vi "Emballage_Lecture_Colonne_Tablebdd.vi"(7 "Where colonne":string[](array[string]), 8 "Error in":errorcluster caption="Error in (no error)", 9 "where valeur":string[](array[string]), 10 "Table":string="configEmballage", 11 "Colonne":string) -> (0 "Error out":errorcluster, 1 "chemin complet":path, 2 "Result Set":string[][](table) caption="Result Set (from first statement with results)", 3 "Column Names":string[](array[string]))   [LabVIEW 2020]
uses:
  Modules/FS/60_FS_Controles/60_FS_SetGet.ctl
  <vilib>/drjdpowell/SQLite Library/SQL Connection/Open (path).vi
  <vilib>/drjdpowell/SQLite Library/SQL Connection/Open (string).vi
  <vilib>/AdvancedString/Path To Command Line String.vi
  <vilib>/drjdpowell/SQLite Library/SQL Connection/Connection.lvclass
panel:
  out "Chaîne":string
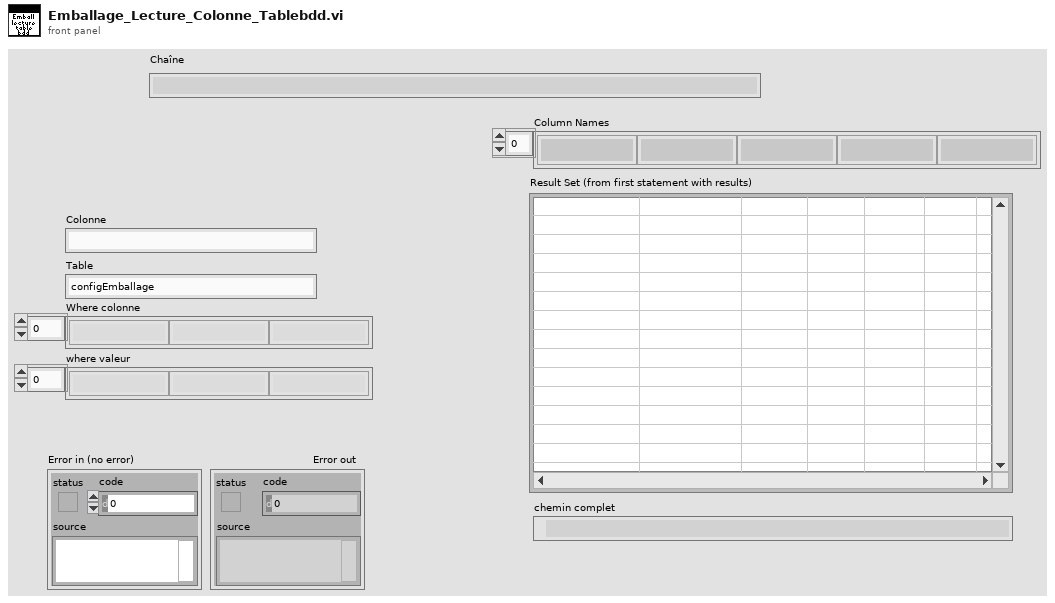
[diagram p1: front panel]
types:
  T1 = typedef "60_FS_SetGet.ctl" = enum16{"set", "get"}
  T2 = typedef "60_FS_CLT_Chemins.ctl" = cluster{"Racine_local":path, "Racine_reseau":path, "Racine_Support_Application":path, "Fichier_Journalisation":path, "Connexion_BDD_VSX":path, "Connexion_BDD_PLZ":path}
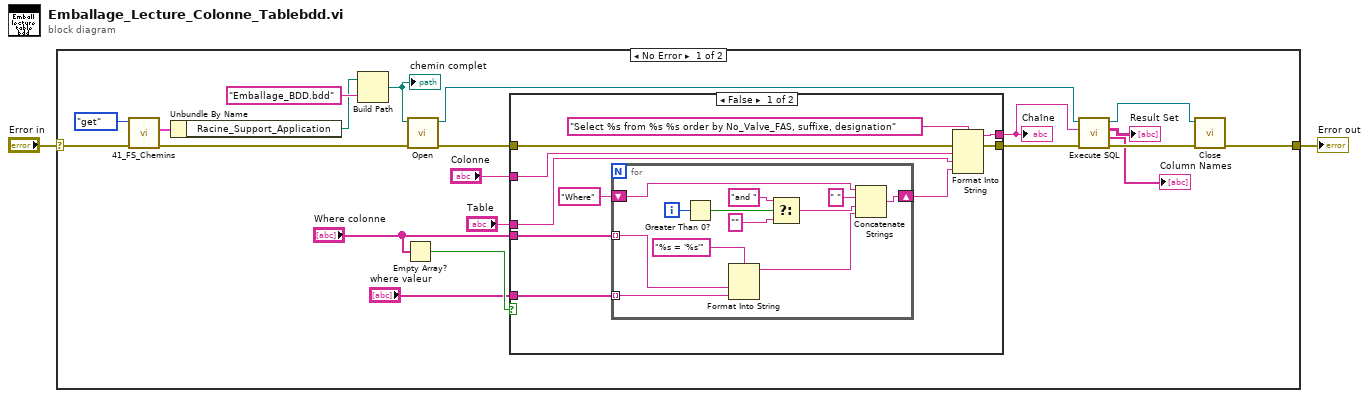
[diagram p0: block diagram]
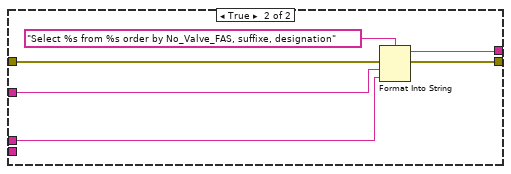
[diagram p2: hidden frame]
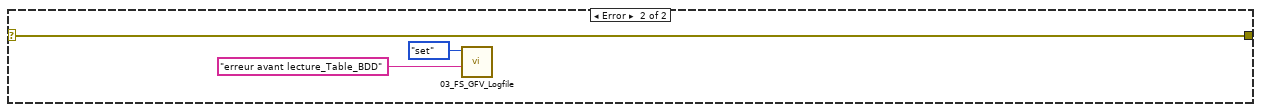
[diagram p3: hidden frame]
diagram:
  n1 = case shown="No Error" "Error in" {
    selector: "Error in" -> [w7 w54]
    tunnel: [w6 w54] -> w1
    frame No Error {
      n2 = call "41_FS_Chemins.vi"("error in (no error)"=w7, "SetGet"=60_FS_SetGet."get") -> ("error out"=w16:errorcluster, "CLT_Chemins_out"=w15:T2)  [unwired: 8 in]
      n3 = Unbundle By Name(w15) -> ("Racine_Support_Application"=w22:path)
      n4 = Build Path(base path=w22, name or relative path="Emballage_BDD.bdd" ("nom ou chemin relatif")) -> (appended path=w21:path)
      "chemin complet" <- w21
      n5 = Empty Array?(array="Where colonne") -> (empty?=w5:bool)
      n6 = call-poly <vilib>:"Open.vi"("error in (no error)"=w16, "db file"=w21) -> ("error out"=w9:errorcluster, "SQLite Connection"=w20:refnum<class "Connection.lvclass">)  [unwired: 8 in]
      n7 = case shown="False" w5 {
        tunnel: [w33 w48] -> w13
        tunnel: "Colonne" -> [w32 w50]
        tunnel: "Table" -> [w31 w49]
        tunnel: w9 -> [w30 w46]
        tunnel: [w29 w47] -> w8
        tunnel: "Where colonne" -> [w25 _]
        tunnel: "where valeur" -> [w24 _]
        frame False {
          n8 = for {
            shift-right: [w44] -> w26
            shift-left: "Where" -> [w45]
            tunnel: w25 -> [w35] mode=indexing
            tunnel: w24 -> [w34] mode=indexing
            i -> [w42]
            n9 = Greater Than 0?(x=w42) -> (x > 0?=w41:bool)
            n10 = Format Into String(format string="%s = '%s'" ("chaîne de format"), w35, w34) -> (resulting string=w36:string)  [unwired: 2 in, 1 out]
            n11 = Select(t="and ", s=w41, f="" ("cas faux")) -> (s? t:f=w40:string)
            n12 = Concatenate Strings(w45, " " ("chaîne"), w40, w36) -> (w44:string)
          }
          n13 = Format Into String(format string="Select %s from %s %s order by No_Valve_FAS, suffixe, designation" ("SQL"), error in=w30, w32, w31, w26) -> (resulting string=w33:string, error out=w29:errorcluster)  [unwired: 1 in]
        }
        frame True {
          n14 = Format Into String(format string="Select %s from %s order by No_Valve_FAS, suffixe, designation" ("SQL"), error in=w46, w50, w49) -> (resulting string=w48:string, error out=w47:errorcluster)  [unwired: 1 in]
        }
      }
      "Chaîne" <- w13
      n15 = call <vilib>:"Execute SQL.vi"("error in (no error)"=w8, "SQL"=w13, "SQLite Connection in"=w20) -> ("error out"=w18:errorcluster, "Column Names"=→"Column Names":string[], "Result Set"=→"Result Set":string[][], "SQLite Connection"=w19:refnum<class "Connection.lvclass">)  [unwired: 5 in]
      n16 = call-dynamic "Close.vi"("error in (no error)"=w18, "SQLite Connection in"=w19) -> ("error out"=w6:errorcluster)  [unwired: 9 in]
    }
    frame Error {
      n17 = call "03_FS_GFV_Logfile.vi"("Chaîne"="erreur avant lecture_Table_BDD", "States"=60_FS_SetGet."set") -> ()  [unwired: 8 in, 2 out]
    }
  }
  "Error out" <- w1
